vi "Requests.vi"(8 "error in (no error)":errorcluster, 9 "write enable":bool=TRUE, 11 "ELAN in":refnum<class "ELAN.lvclass">) -> (0 "error out":errorcluster, 3 "ELAN out":refnum<class "ELAN.lvclass">)   [LabVIEW 2021, in "ELAN.lvclass"]
uses:
  ELAN.lvclass
  D:/my_projects/projects/Algorithms/Labview/21/Master CR/Master CR.lvclass
  Master CR.lvclass/Master CR.ctl
  Network Protocol/Read Network Protocol.vi
  Network Protocol/ELAN Master/ELAN Master.lvclass
  Modbus_v121c/Data Model/Device Data Model.lvclass
  Master CR.lvclass
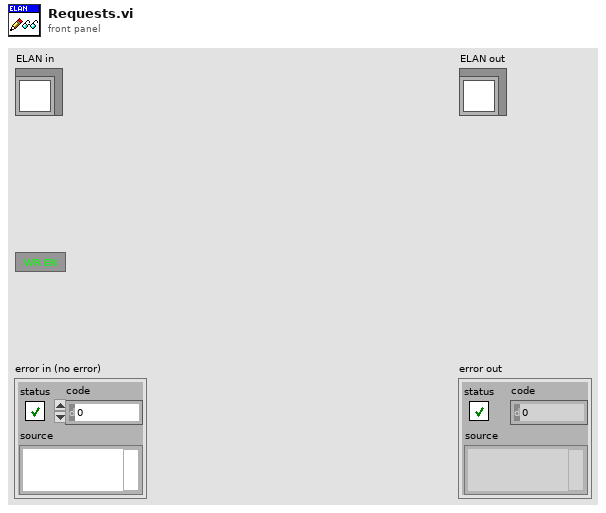
[diagram p1: front panel]
types:
  T1 = typedef "Device Data Model.lvclass/N channel.ctl" = cluster{"N DI channel":i32, "N DO channel":i32, "N AI channel":i32, "N AO channel":i32}
  T2 = typedef "ELAN Data Model.lvclass/Value full.ctl" = cluster{"Value":cluster{"Value":sgl, "units":T3, "component":T4}, "channel state":T5, "collective state":errorcluster}
  T3 = typedef "ELAN PDU.lvclass/Elan units.ctl" = enum16{"Invalid", "no dimension", "ppm", "ppb", "vpm", "ppm C1", "ppm C3", "ppm C6", "mg C/m3", "mg/m3", "%", "% vol", "% of measuring range", "% saturation", "%/°C", "%/K", "% weight", "mV/pH", "mV/mbar", "nA/mbar", "S/m", "S/cm", "mS/m", "mS/cm", "ìS/m", "ìS/cm", "S", "min", "H", "Pa", "MA", "uV", "MV", "V", "mbar", "hPa", "Ml/min", "kOhm", "MOhm", "S1", "°C", "Hz", "pH", "ug/l", "mg/l", "l/min", "uA", "mg/dm3", "kPa", "kOhm*cm", "MOhm*cm", "°", "1/min", "1/m", "g/m3", "g/l", "% Vol C"}
  T4 = typedef "ELAN PDU.lvclass/Elan measured variable.ctl" = enum16{"Invalid", "no component", "CO", "CO2", "CH4 (Methan)", "C6H14 (Hexan)", "SO2", "NO", "NO2", "CHClF2 (R22)", "C3H8 (Propan)", "C4H10 (Butan)", "O2", "C5H12 (Pentan)", "CnHm (THC)", "P (process pressure)", "pH", "T (temperature)", "C2H4 (Ethen)", "C2H2 (Ethin)", "C3H6 (Propen)", "C4H6", "C4H8", "C2H6", "NH3 (Ammoniak)", "N2O", "C6H6 (Benzol)", "SF6", "CH3OH (Methanol)", "C2H5OH (Ethanol)", "CH2Cl2", "C2H4Cl2", "CH3Cl", "C2H4O", "H2O (water vapor)", "G/l (conductivity)", "C", "S", "N", "CF4", "COCl2 (phosgene)", "CHF3 (R23)", "C2F6 (R116)", "------ (self defined component)", "C2H3Cl", "H2 (Hydrogen)", "Ar", "He", "Cl2", "N2"}
  T5 = typedef "ELAN PDU.lvclass/Elan channel state.ctl" = enum16{"Invalid", "Warm-up", "Pause", "Standby", "Measure", "Zero calibration", "Adjust component slope", "Not yet defined1", "Adjust curve dip", "Adjust linearization sensitivity", "Adjust temperature compensation", "Adjust pressure compensation", "Adjust linearization zero", "Not yet defined2", "Autocal", "Adjust phase", "Zero calibration of O2 sensor", "Synchronous zero calibration", "Purging for synchronous zero calibration", "Adjust analog output", "Adjust analog input", "Autocal check"}
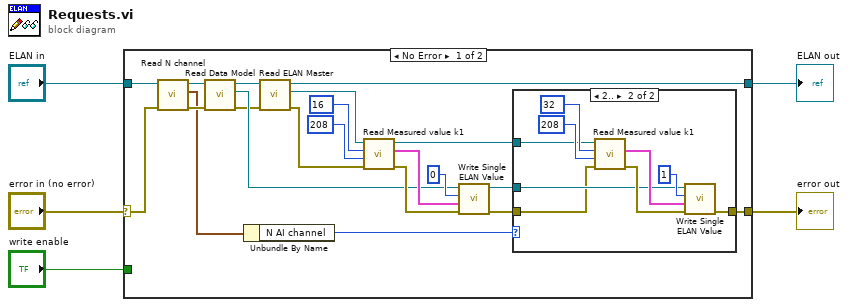
[diagram p0: block diagram]
diagram:
  n1 = case shown="No Error" "error in (no error)" {
    selector: "error in (no error)" -> [w25 w38]
    tunnel: [w11 w38] -> w3
    tunnel: [w17 w37] -> w4
    tunnel: "ELAN in" -> [w26 w37]
    tunnel: "write enable" -> [_ _]
    frame No Error {
      n2 = call "Read N channel.vi"("error in (no error)"=w25, "Master CR in"=w26) -> ("error out"=w20:errorcluster, "N channel"=w7:T1, "Master CR out"=w19:refnum<class "ELAN.lvclass">)  [unwired: 7 in]
      n3 = call "Read Data Model.vi"("error in (no error)"=w20, "Master CR in"=w19) -> ("error out"=w8:errorcluster, "Data Model"=w9:refnum<class "Device Data Model.lvclass">, "Master CR out"=w18:refnum<class "ELAN.lvclass">)  [unwired: 7 in]
      n4 = Unbundle By Name(w7) -> ("N AI channel"=w6:i32)
      n5 = call "Read ELAN Master.vi"("error in (no error)"=w8, "ELAN in"=w18) -> ("error out"=w22:errorcluster, "Network Master"=w12:refnum<class "ELAN Master.lvclass">, "ELAN out"=w17:refnum<class "ELAN.lvclass">)  [unwired: 7 in]
      n6 = call "Read Measured value k1.vi"("error in (no error)"=w22, "Control system address"=u8 208, "Component address"=u8 16, "ELAN master in"=w12) -> ("error out"=w16:errorcluster, "Value"=w15:T2, "ELAN master out"=w10:refnum<class "ELAN Master.lvclass">)  [unwired: 4 in, 1 out]
      n7 = call-dynamic "Write Single ELAN Value.vi"("error in (no error)"=w16, "Value"=w15, "address"=u16 0, "device data model in"=w9) -> ("error out"=w13:errorcluster, "device data model out"=w14:refnum<class "Device Data Model.lvclass">)  [unwired: 6 in]
      n8 = case shown="2.." w6 {
        tunnel: w14 -> [_ w31]
        tunnel: w13 -> [w27 w30]
        tunnel: [w27 w29] -> w11
        tunnel: w10 -> [_ w28]
        frame ..1 {
        }
        frame 2.. {
          n9 = call "Read Measured value k1.vi"("error in (no error)"=w30, "Control system address"=u8 208, "Component address"=u8 32, "ELAN master in"=w28) -> ("error out"=w35:errorcluster, "Value"=w36:T2)  [unwired: 4 in, 2 out]
          n10 = call-dynamic "Write Single ELAN Value.vi"("error in (no error)"=w35, "Value"=w36, "address"=u16 1, "device data model in"=w31) -> ("error out"=w29:errorcluster)  [unwired: 6 in, 1 out]
        }
      }
    }
    frame Error {
    }
  }
  "error out" <- w3
  "ELAN out" <- w4
